vi "Archive Stiffness Jacobian.vi"(8 "error in (no error)":errorcluster, 10 "LBCB Number":T2, 11 "LBCB  Stiffness Jacobian":T3=[[1000000.0, 0.0, 0.0, 0.0, 0.0, 0.0], [0.0, 1000000.0, 0.0, 0.0, 0.0, 0.0], [0.0, 0.0, 1000000.0, 0.0, 0.0, 0.0], [0.0, 0.0, 0.0, 1000000.0, 0.0, 0.0], [0.0, 0.0, 0.0, 0.0, 1000000.0, 0.0], [0.0, 0.0, 0.0, 0.0, 0.0, 1000000.0]]) -> (0 "error out":errorcluster, 2 "String":string)   [LabVIEW 2009]
uses:
  Stiffness Matrix.ctl
  Data Access Objects/Metadata/LBCB Number.ctl
  Dof Names.ctl
panel:
  in  "DOF Names":T1
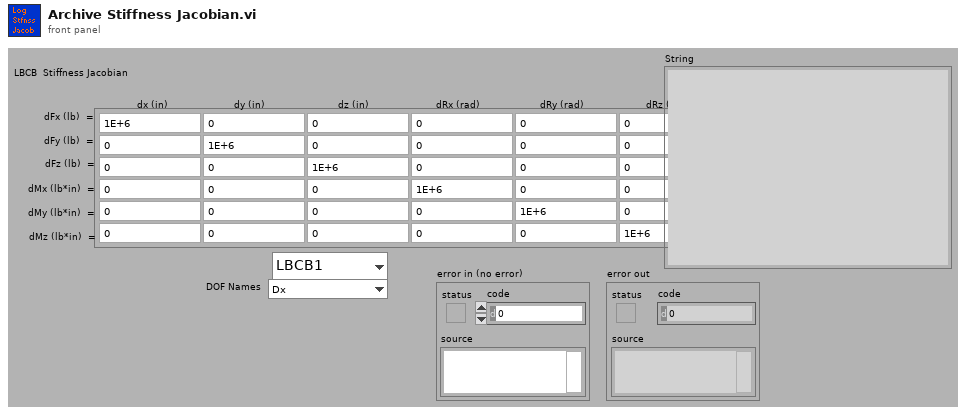
[diagram p1: front panel]
types:
  T1 = typedef "Dof Names.ctl" = enum16{"Dx", "Dy", "Dz", "Rx", "Ry", "Rz", "Fx", "Fy", "Fz", "Mx", "My", "Mz"}
  T2 = typedef "LBCB Number.ctl" = enum16{"LBCB1", "LBCB2"}
  T3 = typedef "Stiffness Matrix.ctl" = dbl[][]
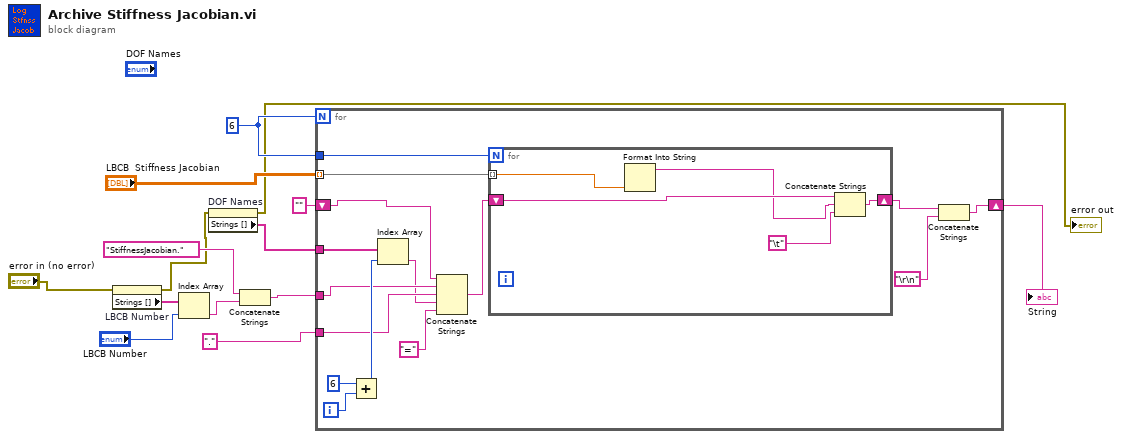
[diagram p0: block diagram]
diagram:
  w14 = 6
  n1 = property on="LBCB Number" class="Enum (strict)"(error in="error in (no error)") -> (error out=w4:errorcluster, "Strings []"=w13:string[])  [unwired: 1 in, 1 out]
  n2 = Index Array(array=w13, index="LBCB Number") -> (element=w11:string)
  n3 = property on="DOF Names" class="Enum (strict)"(error in=w4) -> (error out=→"error out":errorcluster, "Strings []"=w7:string[])  [unwired: 1 in, 1 out]
  n4 = Concatenate Strings("StiffnessJacobian.", w11) -> (w8:string)
  n5 = for {
    N: w14 -> [_]
    tunnel: w14 -> [w29]
    tunnel: "LBCB  Stiffness Jacobian" -> [w28] mode=indexing
    tunnel: w8 -> [w21]
    tunnel: w7 -> [w24]
    tunnel: "." ("element") -> [w23]
    shift-right: [w18] -> w5
    shift-left: "" -> [w16]
    i -> [w27]
    n6 = Add(x=6, y=w27) -> (x+y=w25:i32)
    n7 = Index Array(array=w24, index=w25) -> (element=w20:string)
    n8 = Concatenate Strings(w16, w21, w23, w20, "=" ("string")) -> (w15:string)
    n9 = for {
      N: w29 -> [_]
      tunnel: w28 -> [w34] mode=indexing
      shift-right: [w33] -> w22
      shift-left: w15 -> [w32]
      n10 = Format Into String(w34) -> (resulting string=w31:string)  [unwired: 3 in, 1 out]
      n11 = Concatenate Strings(w32, w31, "\t") -> (w33:string)
    }
    n12 = Concatenate Strings(w22, "\r\n") -> (w18:string)
  }
  "String" <- w5
